vi "Coerce Position.vi"(8 "Robot Pos In":cluster{dbl, dbl}, 10 "Robot Pos Before Shmoove":cluster{dbl, dbl}, 11 "Blue Side?":bool) -> (0 "Robot Pos Out":cluster{dbl, dbl})   [LabVIEW 2025]
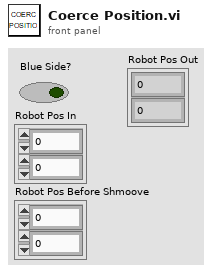
[diagram p1: front panel]
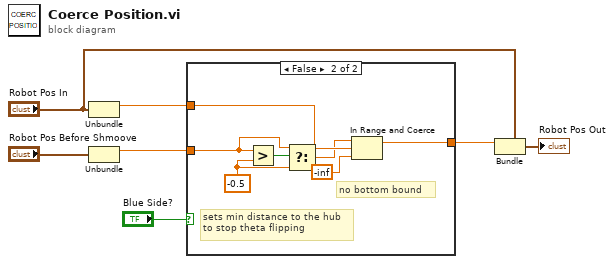
[diagram p0: block diagram]
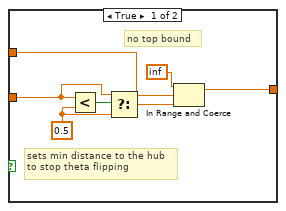
[diagram p2: hidden frame]
diagram:
  n1 = Unbundle("Robot Pos In") -> (w2:dbl)  [unwired: 1 out]
  n2 = Unbundle("Robot Pos Before Shmoove") -> (w3:dbl)  [unwired: 1 out]
  n3 = case shown="False" "Blue Side?" {
    tunnel: w3 -> [w12 w19]
    tunnel: w2 -> [w9 w18]
    tunnel: [w8 w17] -> w1
    frame True {
      w13 = 0.5 ("y")
      # "no top bound"
      # "sets min distance to the hub\nto stop theta flipping"
      n4 = Less?(x=w12, y=w13) -> (x < y?=w14:bool)
      n5 = Select(t=w12, s=w14, f=w13) -> (s? t:f=w11:dbl)
      n6 = In Range and Coerce(upper limit=inf, x=w9, lower limit=w11) -> (coerced(x)=w8:dbl)  [unwired: 1 out]
    }
    frame False {
      w20 = -0.5 ("y")
      # "no bottom bound"
      # "sets min distance to the hub\nto stop theta flipping"
      n7 = Greater?(x=w19, y=w20) -> (0:w21:bool)
      n8 = Select(t=w19, s=w21, f=w20) -> (s? t:f=w16:dbl)
      n9 = In Range and Coerce(upper limit=w16, x=w18, lower limit=-inf) -> (coerced(x)=w17:dbl)  [unwired: 1 out]
    }
  }
  n10 = Bundle(cluster="Robot Pos In", w1) -> (→"Robot Pos Out":cluster{dbl, dbl})  [unwired: 1 in]
